vi "Write App INI.vi"(6 "Node":string, 8 "error in (no error)":errorcluster, 9 "Cluster":string, 10 "System":string, 11 "System Config Module in":refnum<class "System Config Module.lvclass">) -> (0 "error out":errorcluster, 2 "Main Config Path":path, 3 "System Config Module out":refnum<class "System Config Module.lvclass">, 4 "INI Path":path)   [LabVIEW 2020, in "Volatus.lvlib" / "System Config Module.lvclass"]
uses:
  System Config Module.lvclass
  System Config Module.lvclass/System Config Module.ctl
  <vilib>/Utility/config.llb/Write Key (String).vi
  <vilib>/Utility/config.llb/Read Key (String).vi
  Volatus.lvlib
  <vilib>/Utility/config.llb/NI_LVConfig.lvlib
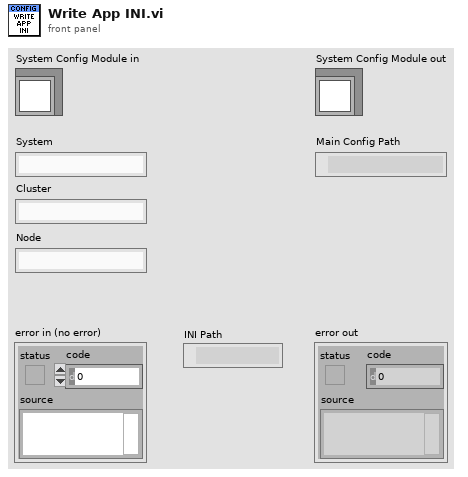
[diagram p1: front panel]
types:
  T1 = typedef "NI_LVConfig.lvlib/Config Data RefNum.ctl" = refnum<k1>
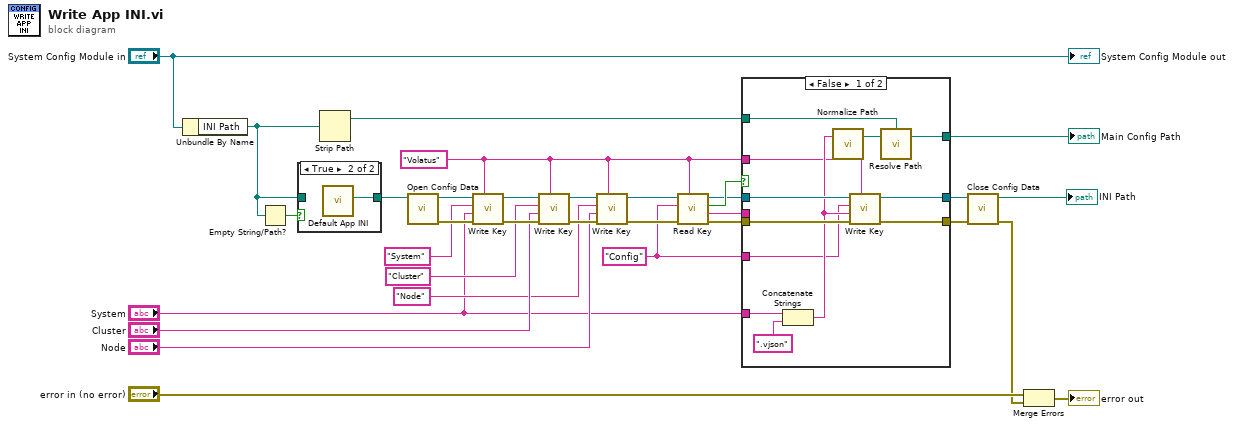
[diagram p0: block diagram]
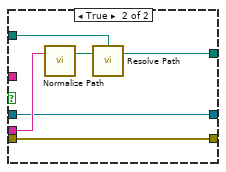
[diagram p2: hidden frame]
diagram:
  w6 = "Config"
  w13 = "Volatus" ("section")
  n1 = Unbundle By Name("System Config Module in") -> ("INI Path"=w10:path)
  n2 = Empty String/Path?(string/path=w10) -> (empty?=w30:bool)
  n3 = case shown="True" w30 {
    tunnel: w10 -> [w33 _]
    tunnel: [w33 w34] -> w29
    frame False {
    }
    frame True {
      n4 = call "Default App INI.vi"() -> ("Default App INI"=w34:path)  [unwired: 11 in]
    }
  }
  n5 = Strip Path(path=w10) -> (stripped path=w9:path)  [unwired: 1 out]
  n6 = call <vilib>:"Open Config Data.vi"("configuration file path"=w29) -> ("error out"=w21:errorcluster, "refnum"=w28:T1)  [unwired: 8 in, 1 out]
  n7 = call-poly <vilib>:"Write Key.vi"("section"=w13, "error in (no error)"=w21, "value"="System", "key"="System", "refnum"=w28) -> ("error out"=w22:errorcluster, "refnum out"=w27:T1)  [unwired: 4 in, 1 out]
  n8 = call-poly <vilib>:"Write Key.vi"("section"=w13, "error in (no error)"=w22, "value"="Cluster", "key"="Cluster", "refnum"=w27) -> ("error out"=w23:errorcluster, "refnum out"=w26:T1)  [unwired: 4 in, 1 out]
  n9 = call-poly <vilib>:"Write Key.vi"("section"=w13, "error in (no error)"=w23, "value"="Node", "key"="Node", "refnum"=w26) -> ("error out"=w24:errorcluster, "refnum out"=w25:T1)  [unwired: 4 in, 1 out]
  n10 = call-poly <vilib>:"Read Key.vi"("section"=w13, "error in (no error)"=w24, "key"=w6, "refnum"=w25) -> ("error out"=w12:errorcluster, "value"=w11:string, "found?"=w15:bool, "refnum out"=w14:T1)  [unwired: 4 in]
  n11 = case shown="False" w15 {
    tunnel: w14 -> [w41 w48]
    tunnel: w13 -> [w38 _]
    tunnel: w12 -> [w40 w47]
    tunnel: w11 -> [_ w51]
    tunnel: w9 -> [w43 w50]
    tunnel: [w42 w49] -> w8
    tunnel: "System" -> [w45 _]
    tunnel: w6 -> [w37 _]
    tunnel: [w36 w48] -> w5
    tunnel: [w35 w47] -> w4
    frame False {
      n12 = Concatenate Strings(w45, ".vjson" ("string")) -> (w39:string)
      n13 = call "Normalize Path.vi"("Path String"=w39) -> ("Path"=w46:path)  [unwired: 2 in]
      n14 = call-poly <vilib>:"Write Key.vi"("section"=w38, "error in (no error)"=w40, "value"=w39, "key"=w37, "refnum"=w41) -> ("error out"=w35:errorcluster, "refnum out"=w36:T1)  [unwired: 4 in, 1 out]
      n15 = call "Resolve Path.vi"("Starting Path"=w43, "Path"=w46) -> ("Resolved Path"=w42:path)  [unwired: 4 in]
    }
    frame True {
      n16 = call "Normalize Path.vi"("Path String"=w51) -> ("Path"=w52:path)  [unwired: 2 in]
      n17 = call "Resolve Path.vi"("Starting Path"=w50, "Path"=w52) -> ("Resolved Path"=w49:path)  [unwired: 4 in]
    }
  }
  "Main Config Path" <- w8
  n18 = call <vilib>:"Close Config Data.vi"("error in (no error)"=w4, "refnum"=w5) -> ("error out"=w2:errorcluster, "file path"=→"INI Path":path)  [unwired: 8 in]
  n19 = Merge Errors("error in (no error)", w2) -> (→"error out":errorcluster)
  "System Config Module out" <- "System Config Module in"
